vi "IMPRIMER ETIQUETTE EMBALLAGE SIMPLE.vi"() -> ()   [LabVIEW 2013]
panel:
  in  "indice client":string="03"
  in  "N°article client":string="EL-360"
  in  "Société de facturation":string(combo)="Fluid Automation Systems SA"
  in  "Affiche code bar client":string(combo)="OUI"
  in  "n° commande FAS":string="03838/08-07.01.01"
  out "Ref client":string="EL-360 "
  in  "Langue":string(combo)="ANG"
  out "nom sous code bar client":string="EL-360  03 25 "
  in  "destinataire":string="EMS Electro Medical System"
  in  "n° cmde client":string="CF-08-0253/2"
  in  "Quantité":string="25/100"
  in  "carton":string="1/4"
  in  "nom valve FAS":string="12-216C-04520 EQIFIL 104mA 36ohm"
  out "chaine  à écrire":string="ZB\nUS\nq592\nD7\nN\nR166,48\nI8,12,001\rA504,828,2,1,1,1,N,\"fluid automation systems sa\"\nA504,812,2,1,1,1,N,\"route del'Etraz 126 CP 256\"\nA504,796,2,1,1,1,N,\"CH-1290 Versoix\"\nA504,780,2,1,1,1,N,\"Tl.+41(0)22 775 10 01\"\nA504,764,2,1,1,1,N,\"www.fas.ch\"\rGW0,824,67,55,ÿÿÿÿÿÿÿÿÿÿÿÿÿÿÿÿÿÿÿÿÿÿÿÿÿÿÿÿÿÿÿÿÿÿÿÿÿÿÿÿÿÿÿÿÿÿÿÿÿÿÿÿÿÿÿÿÿÿÿÿÿÿÿÿÿáÿÿÿÿÿÿÿÿÿÿÿÿÿÿÿÿÿÿÿÿÿÿÿÿÿÿÿÿÿÿÿÿÿÿÿÿÿÿÿÿÿÿÿÿÿÿÿÿÿÿÿÿÿÿÿÿÿÿÿÿÿÿÿÿÿÿÿÿÿÿÿÿÿÿÿÿÿÿÿÿÿÿÿÀÿÿÿÿÿÿÿÿÿÿÿÿÿÿÿÿÿÿÿÿÿÿÿÿÿÿÿÿÿÿÿÿÿÿÿÿÿÿÿÿÿÿÿÿÿÿþ\u0000ÿÿÿÿÿÿÿÿÿÿÿÿÿÿÿÿÿ\u0000ÿÿÿÿÿÿÿÿÿÿÿÿÿÿÿÿÿÿÿÿÿÿÿÿÿÿÿÿÿÿÿÿÿÿÿÿÿÿÿÿÿÿÿÿÿÿø\u0000ÿÿÿÿÿÿÿÿÿÿÿÿÿÿÿÿþ\u0000ÿÿÿÿÿÿÿÿÿÿÿÿÿÿÿÿÿÿÿÿÿÿÿÿÿÿÿÿÿÿÿÿÿÿÿÿÿÿÿÿÿÿÿÿÿÿð\u0000ÿÿÿÿÿÿÿ..."
  # "Destinataire:"
  # "N°commande :"
  # "Carton :"
  # "Quantité:"
  # "Votre ref.:"
  # "FASmedic s.a.\nZone industrielle\nCH-1607 Palézieux-Gare\nTél.+41(0)21 907 79 71\nwww.fasmedic.com"
  # "N°article FAS:"
  # "N°commande FAS:"
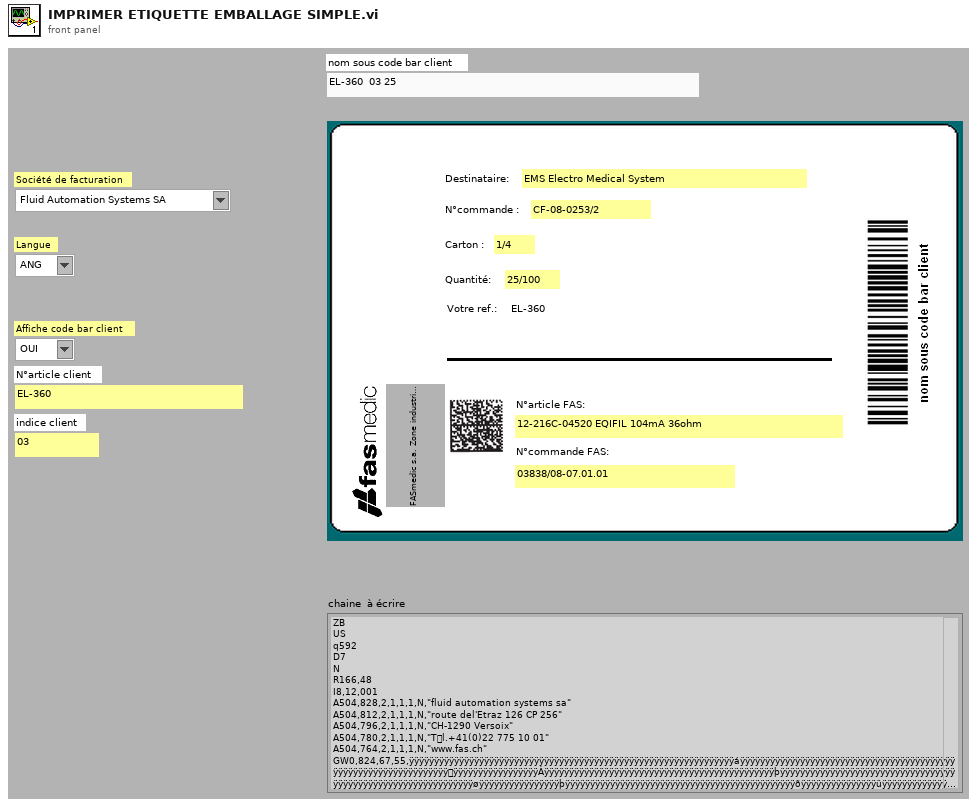
[diagram p1: front panel]
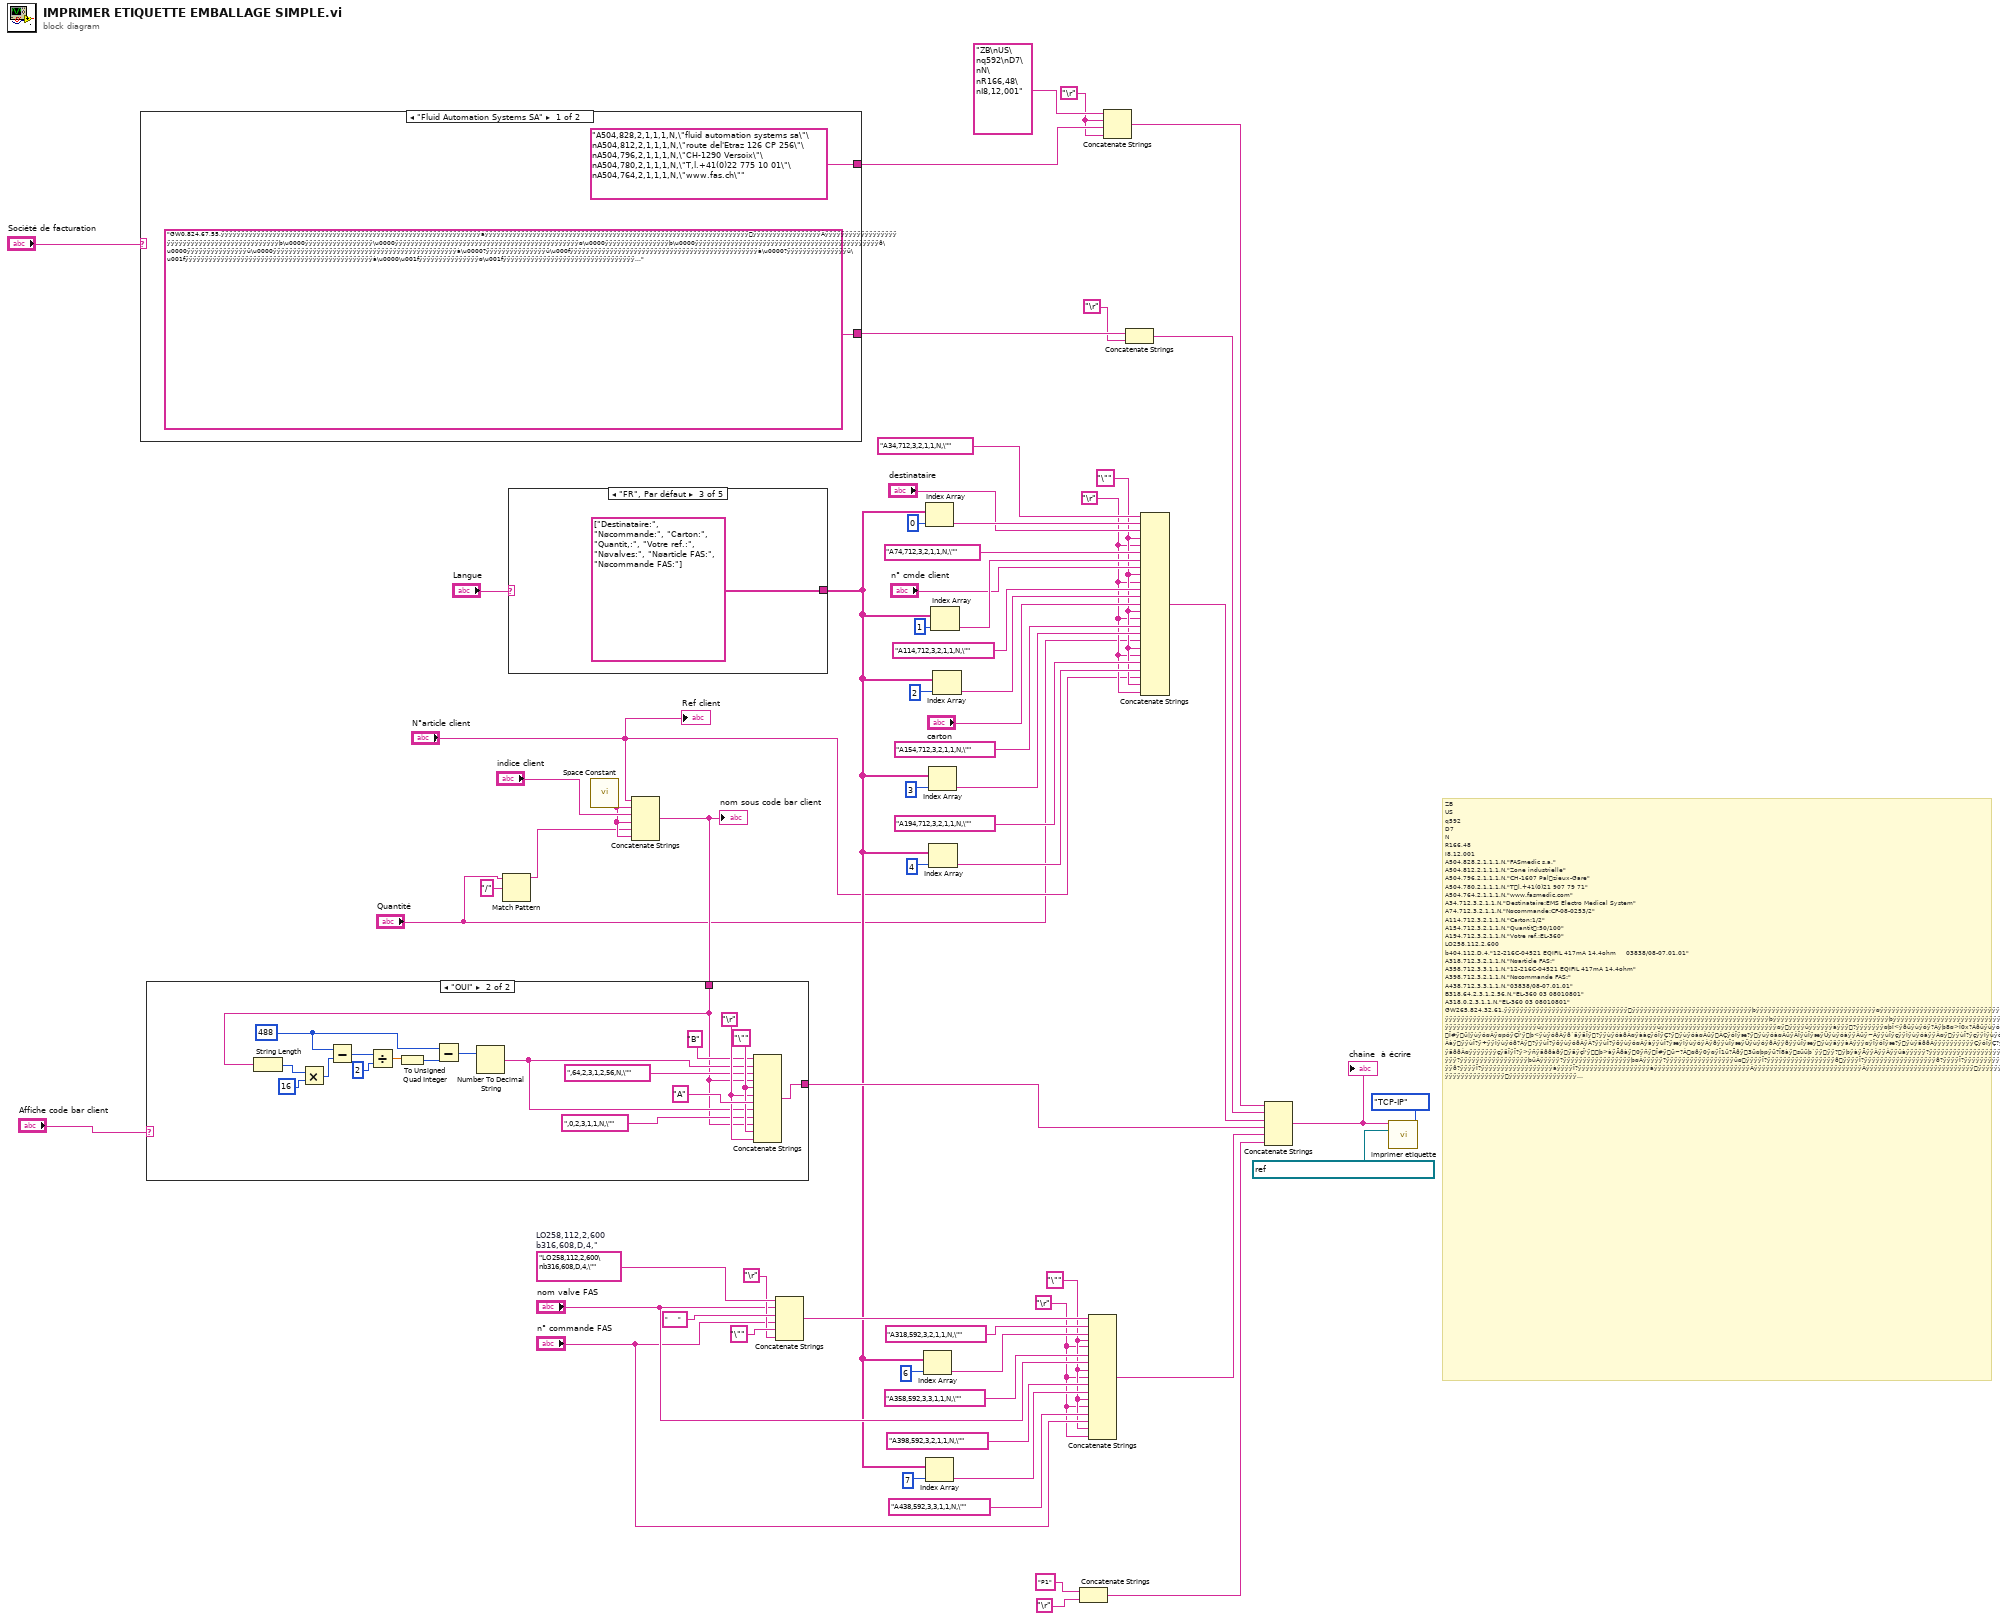
[diagram p0: block diagram]
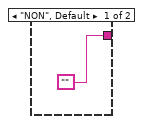
[diagram p2: hidden frame]
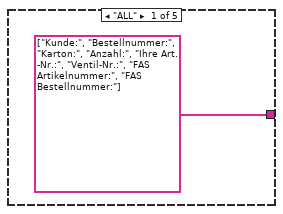
[diagram p3: hidden frame]
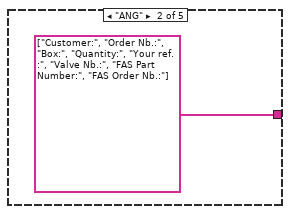
[diagram p4: hidden frame]
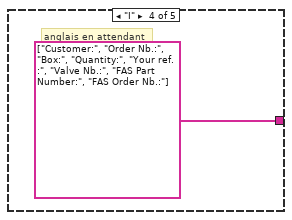
[diagram p5: hidden frame]
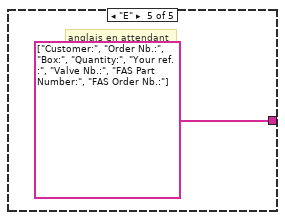
[diagram p6: hidden frame]
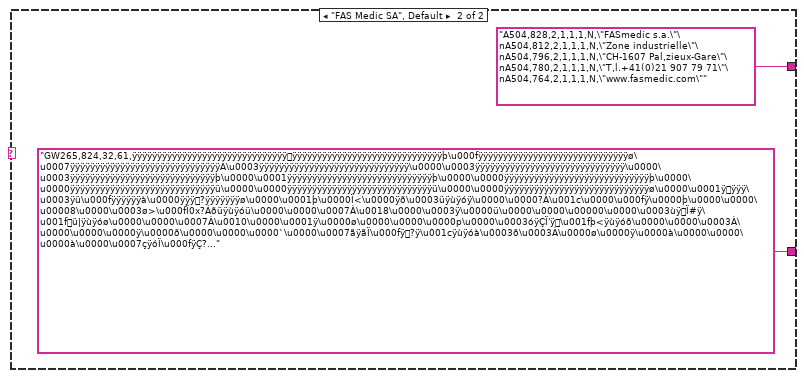
[diagram p7: hidden frame]
diagram:
  w22 = "\r"
  w23 = "\""
  w38 = "LO258,112,2,600\nb316,608,D,4,\""  # LO258,112,2,600 b316,608,D,4,"
  w40 = "\""
  w39 = "\r"
  w59 = "\r"
  # "ZB\nUS\nq592\nD7\nN\nR166,48\nI8,12,001\nA504,828,2,1,1,1,N,\"FASmedic s.a.\"\nA504,812,2,1,1,1,N,\"Zone industrielle\"\nA504,796,2,1,1,1,N,\"CH-1607 Palzieux-Gare\"\nA504,780,2,1,1,1,N,\"Tl.+41(0)21 907 79 71\"\nA504,764,2,1,1,1,N,\"www.fasmedic.com\"\nA34,712,3,2,1,1,N,\"Destinataire:EMS Electro Medical System\"\nA74,712,3,2,1,1,N,\"Nøcommande:CF-08-0253/2\"\nA114,712,3,2,1,1,N,\"Carton:1/2\"\nA154,712,3,2,1,1,N,\"Quantit:50/100\"\nA194,712,3,2,1,1,N,\"Votre ref.:EL-360\"\nLO258,112,2,600\nb404,112,D,4,\"12-216C-04521 EQIFIL 417mA 14.4ohm     03838/08-07.01.01\"\nA318,712,3,2,1,1,N,\"Nøarticle FAS:\"\nA358,712,3,3,1,1,N,\"12-216C-04521 EQIFIL 417mA 14.4ohm\"\nA398,712,3,2,1,1,N,\"Nøcommande FAS:\"\nA438,712,3,3,1,1,N,\"03838/08-07.01.01\"\nB318,64,2,3,1,2,56,N,\"EL-360 03 08010801\"\nA318,0,2,3,1,1,N,\"EL-360 03 08010801\"\nGW265,824,32,61,ÿÿ..."
  n1 = case shown="\"Fluid Automation Systems SA\"" "Société de facturation" {
    tunnel: ["GW0,824,67,55,ÿÿÿÿÿÿÿÿÿÿÿÿÿÿÿÿÿÿÿÿÿÿÿÿÿÿÿÿÿÿÿÿÿÿÿÿÿÿÿÿÿÿÿÿÿÿÿÿÿÿÿÿÿÿÿÿÿÿÿÿÿÿÿÿÿáÿÿÿÿÿÿÿÿÿÿÿÿÿÿÿÿÿÿÿÿÿÿÿÿÿÿÿÿÿÿÿÿÿÿÿÿÿÿÿÿÿÿÿÿÿÿÿÿÿÿÿÿÿÿÿÿÿÿÿÿÿÿÿÿÿÿÿÿÿÿÿÿÿÿÿÿÿÿÿÿÿÿÿÀÿÿÿÿÿÿÿÿÿÿÿÿÿÿÿÿÿÿÿÿÿÿÿÿÿÿÿÿÿÿÿÿÿÿÿÿÿÿÿÿÿÿÿÿÿÿþ\u0000ÿÿÿÿÿÿÿÿÿÿÿÿÿÿÿÿÿ\u0000ÿÿÿÿÿÿÿÿÿÿÿÿÿÿÿÿÿÿÿÿÿÿÿÿÿÿÿÿÿÿÿÿÿÿÿÿÿÿÿÿÿÿÿÿÿÿø\u0000ÿÿÿÿÿÿÿÿÿÿÿÿÿÿÿÿþ\u0000ÿÿÿÿÿÿÿÿÿÿÿÿÿÿÿÿÿÿÿÿÿÿÿÿÿÿÿÿÿÿÿÿÿÿÿÿÿÿÿÿÿÿÿÿÿÿð\u0000ÿÿÿÿÿÿÿÿÿÿÿÿÿÿÿü\u0000ÿÿÿÿÿÿÿÿÿÿÿÿÿÿÿÿÿÿÿÿÿÿÿÿÿÿÿÿÿÿÿÿÿÿÿÿÿÿÿÿÿÿÿÿÿÿà\u0000?ÿÿÿÿÿÿÿÿÿÿÿÿÿÿÿü\u000fÿÿÿÿÿÿÿÿÿÿÿÿÿÿÿÿÿÿÿÿÿÿÿÿÿÿÿÿÿÿÿÿÿÿÿÿÿÿÿÿÿÿÿÿÿÿÿà\u0000?ÿÿÿÿÿÿÿÿÿÿÿÿÿÿÿü\u001fÿÿÿÿÿÿÿÿÿÿÿÿÿÿÿÿÿÿÿÿÿÿÿÿÿÿÿÿÿÿÿÿÿÿÿÿÿÿÿÿÿÿÿÿÿÿÿà\u0000\u001fÿÿÿÿÿÿÿÿÿÿÿÿÿÿÿø\u001fÿÿÿÿÿÿÿÿÿÿÿÿÿÿÿÿÿÿÿÿÿÿÿÿÿÿÿÿÿÿÿÿÿ..." "GW265,824,32,61,ÿÿÿÿÿÿÿÿÿÿÿÿÿÿÿÿÿÿÿÿÿÿÿÿÿÿÿÿÿÿÿÿÿÿÿÿÿÿÿÿÿÿÿÿÿÿÿÿÿÿÿÿÿÿÿÿÿÿÿÿÿþ\u000fÿÿÿÿÿÿÿÿÿÿÿÿÿÿÿÿÿÿÿÿÿÿÿÿÿÿÿÿÿÿø\u0007ÿÿÿÿÿÿÿÿÿÿÿÿÿÿÿÿÿÿÿÿÿÿÿÿÿÿÿÿÿÿÀ\u0003ÿÿÿÿÿÿÿÿÿÿÿÿÿÿÿÿÿÿÿÿÿÿÿÿÿÿÿÿÿÿ\u0000\u0003ÿÿÿÿÿÿÿÿÿÿÿÿÿÿÿÿÿÿÿÿÿÿÿÿÿÿÿÿÿÿ\u0000\u0003ÿÿÿÿÿÿÿÿÿÿÿÿÿÿÿÿÿÿÿÿÿÿÿÿÿÿÿÿÿþ\u0000\u0001ÿÿÿÿÿÿÿÿÿÿÿÿÿÿÿÿÿÿÿÿÿÿÿÿÿÿÿÿÿþ\u0000\u0000ÿÿÿÿÿÿÿÿÿÿÿÿÿÿÿÿÿÿÿÿÿÿÿÿÿÿÿÿÿþ\u0000\u0000ÿÿÿÿÿÿÿÿÿÿÿÿÿÿÿÿÿÿÿÿÿÿÿÿÿÿÿÿÿü\u0000\u0000ÿÿÿÿÿÿÿÿÿÿÿÿÿÿÿÿÿÿÿÿÿÿÿÿÿÿÿÿÿü\u0000\u0000ÿÿÿÿÿÿÿÿÿÿÿÿÿÿÿÿÿÿÿÿÿÿÿÿÿÿÿÿÿø\u0000\u0001ÿÿÿÿ\u0003ÿü\u000fÿÿÿÿÿÿà\u0000ÿÿÿ?ÿÿÿÿÿÿÿø\u0000\u0001þ\u0000Ï<\u0000ÿð\u0003üÿùÿóÿ\u0000\u0000?À\u001c\u0000\u000fÿ\u0000þ\u0000\u0000\u00008\u0000\u0003ø>\u000fÏ0x?Áðüÿùÿóü\u0000\u0000\u0007À\u0018\u0000\u0003ÿ\u0000ü\u0000\u0000\u00000\u0000\u0003ùÿÏ#ÿ\u001fü|ÿùÿóø\u0000\u0000\u0007À\u0010\u0000\u0001ÿ\u0000ø\u0000\u0000\u0000p\u0000\u0003óÿÇÏ'ÿ\u001fþ<ÿùÿóð\u0000\u0000\u0003À\u0000\u0000\u0000ÿ\u0000ð\u0000\u0000\u0000`\u0000\u0007ãÿãÏ\u000fÿ?ÿ\u001cÿùÿóà\u0003ð\u0003À\u0000ø\u0000ÿ\u0000à\u0000\u0000\u0000à\u0000\u0007çÿóÏ\u000fÿÇ?..."] -> w18
    tunnel: ["A504,828,2,1,1,1,N,\"fluid automation systems sa\"\nA504,812,2,1,1,1,N,\"route del'Etraz 126 CP 256\"\nA504,796,2,1,1,1,N,\"CH-1290 Versoix\"\nA504,780,2,1,1,1,N,\"T‚l.+41(0)22 775 10 01\"\nA504,764,2,1,1,1,N,\"www.fas.ch\"" "A504,828,2,1,1,1,N,\"FASmedic s.a.\"\nA504,812,2,1,1,1,N,\"Zone industrielle\"\nA504,796,2,1,1,1,N,\"CH-1607 Pal‚zieux-Gare\"\nA504,780,2,1,1,1,N,\"T‚l.+41(0)21 907 79 71\"\nA504,764,2,1,1,1,N,\"www.fasmedic.com\""] -> w60
    frame "Fluid Automation Systems SA" {
    }
    frame "FAS Medic SA", Default {
    }
  }
  n2 = Match Pattern(string="Quantité", regular expression="/" ("expression régulière")) -> (before substring=w3:string)  [unwired: 1 in, 3 out]
  n3 = case shown="\"FR\", Par défaut" "Langue" {
    tunnel: [string[] ["Kunde:", "Bestellnummer:", "Karton:", "Anzahl:", "Ihre Art.-Nr.:", "Ventil-Nr.:", "FAS Artikelnummer:", "FAS Bestellnummer:"] string[] ["Customer:", "Order Nb.:", "Box:", "Quantity:", "Your ref.:", "Valve Nb.:", "FAS Part Number:", "FAS Order Nb.:"] string[] ["Destinataire:", "Nøcommande:", "Carton:", "Quantit‚:", "Votre ref.:", "Nøvalves:", "Nøarticle FAS:", "Nøcommande FAS:"] string[] ["Customer:", "Order Nb.:", "Box:", "Quantity:", "Your ref.:", "Valve Nb.:", "FAS Part Number:", "FAS Order Nb.:"] string[] ["Customer:", "Order Nb.:", "Box:", "Quantity:", "Your ref.:", "Valve Nb.:", "FAS Part Number:", "FAS Order Nb.:"]] -> w9
    frame "ALL" {
    }
    frame "ANG" {
    }
    frame "FR", Default {
    }
    frame "I" {
      # "anglais en attendant"
    }
    frame "E" {
      # "anglais en attendant"
    }
  }
  n4 = call <vilib>:"Space Constant.vi"() -> ("String"=w7:string)
  n5 = Concatenate Strings("N°article client", w7, "indice client", w7, w3, w7) -> (w21:string)
  "nom sous code bar client" <- w21
  n6 = case shown="\"OUI\"" "Affiche code bar client" {
    tunnel: w21 -> [_ w75]
    tunnel: ["" w89] -> w13
    frame "NON", Default {
    }
    frame "OUI" {
      w83 = 488
      w91 = "\""
      w90 = "\r"
      n7 = String Length(string=w75) -> (length=w88:i32)
      n8 = Multiply(x=w88, y=16) -> (x*y=w86:i32)
      n9 = Subtract(x=w83, y=w86) -> (x-y=w85:i32)
      n10 = Divide(x=w85, y=2) -> (x/y=w82:dbl)
      n11 = To Unsigned Quad Integer(1:w82) -> (0:w81:u64)
      n12 = Subtract(x=w83, y=w81) -> (x-y=w80:u64)
      n13 = Number To Decimal String(number=w80) -> (decimal integer string=w76:string)  [unwired: 1 in]
      n14 = Concatenate Strings("B", w76, ",64,2,3,1,2,56,N,\"", w75, w91, w90, "A", w76, ",0,2,3,1,1,N,\"", w75, w91, w90) -> (w89:string)
    }
  }
  n15 = Concatenate Strings(w38, "nom valve FAS", "     ", "n° commande FAS", "\"", "\r") -> (w32:string)
  n16 = Index Array(array=w9, index=6 ("indice")) -> (element=w30:string)
  n17 = Index Array(array=w9, index=0 ("indice")) -> (element=w56:string)
  n18 = Index Array(array=w9, index=7 ("indice")) -> (element=w26:string)
  n19 = Index Array(array=w9, index=3 ("indice")) -> (element=w44:string)
  n20 = Index Array(array=w9, index=4 ("indice")) -> (element=w42:string)
  n21 = Index Array(array=w9, index=1 ("indice")) -> (element=w52:string)
  n22 = Index Array(array=w9, index=2 ("indice")) -> (element=w48:string)
  n23 = Concatenate Strings("P1", "\r") -> (w11:string)
  n24 = Concatenate Strings(w32, "A318,592,3,2,1,1,N,\"", w30, w23, w22, "A358,592,3,3,1,1,N,\"", "nom valve FAS", w23, w22, "A398,592,3,2,1,1,N,\"", w26, w23, w22, "A438,592,3,3,1,1,N,\"", "n° commande FAS", w23, w22) -> (w12:string)
  n25 = Concatenate Strings("ZB\nUS\nq592\nD7\nN\nR166,48\nI8,12,001", w59, w60, w59) -> (w16:string)
  n26 = Concatenate Strings(w18, "\r") -> (w15:string)
  n27 = Concatenate Strings("A34,712,3,2,1,1,N,\"", w56, "destinataire", w40, w39, "A74,712,3,2,1,1,N,\"", w52, "n° cmde client", w40, w39, "A114,712,3,2,1,1,N,\"", w48, "carton", w40, w39, "A154,712,3,2,1,1,N,\"", w44, "Quantité", w40, w39, "A194,712,3,2,1,1,N,\"", w42, "N°article client", w40, w39) -> (w14:string)
  n28 = Concatenate Strings(w16, w15, w14, w13, w12, w11) -> (w10:string)
  "chaine  à écrire" <- w10
  n29 = call "imprimer etiquette.vi"("chaine à écrire"=w10, "Type de liaison"=enum16{"RS232", "USB", "TCP-IP", "Aucune"}."TCP-IP", "Nom de ressource VISA TCP-IP"=refnum<visa-resource-name> "TCPIP0::10.41.9.129::9100::socket") -> ()  [unwired: 12 in, 1 out]
  "Ref client" <- "N°article client"
